vi "GL_controller.VI"(0 "Motion Settings":T1={"No Motion?"=FALSE, "Motion System"=enum."NI 735x", "Motion Bd ID"=1, "Motion Profile"="SMAC1", "# Axis"=1, "Reverse Z axis?"=TRUE, "SMAC Axis"=0, "scan pair"=enum."y-(x) scan", "RT fps"=6.0, "Steps per mm"=[1000, 1000, 1000, 1000], "Motor Parameters"={"velocity ct/s"=[10000.0, 10000.0, 10000.0, 50000.0], "accel ct/s^2"=[50000.0, 50000.0, 50000.0, 200000.0]}, "One Way Scan"=FALSE, "Reverse One Way Scan"=FALSE, "Global Position (mm)"=[], "Plane"=0, "Distance between\nscan lines (um)"=0.0, "Distance between\nscan planes (um)"=0.0, "number of scan planes"=1, "Total steps in line"=0, "Xtra plane\ndistance  (um)"=100, "Xtra planes "=1, "Add Axis"=FALSE, "overshoot cts"=200, "BKPT Shift"=0, "Scan Start Time (ms)"=0, "ESP VISA"="GPIB::1::INSTR", "3rd Axis"=1, "GL Ref Out"=refnum, "Galil Address"=""} {"3rd Axis" items=["x", "y", "z", "w"]; "Xtra planes" min=1; "Xtra plane\ndistance  (um)" min=0; "Distance between\nscan planes (um)" format="%.2f"; "Distance between\nscan lines (um)" format="%.2f"; "SMAC Axis" items=["None"=0, "Axis 1"=1, "Axis 2"=2, "Axis 3"=3, "Axis 4"=4, "Axis 5"=5, "Axis 6"=6, "Axis 7"=7, "Axis 8"=8, "Vector Space 1"=17, "Vector Space 2"=18, "Vector Space 3"=19, "Vector Space 4"=20]; "Motion Bd ID" min=1 max=32 step=1}, 4 "Initialize":bool=TRUE) -> (5 "Motion Settings Out":T1={"No Motion?"=FALSE, "Motion System"=enum."NI 735x", "Motion Bd ID"=1, "Motion Profile"="SMAC1", "# Axis"=1, "Reverse Z axis?"=TRUE, "SMAC Axis"=0, "scan pair"=enum."y-(x) scan", "RT fps"=6.0, "Steps per mm"=[1000, 1000, 1000, 1000], "Motor Parameters"={"velocity ct/s"=[10000.0, 10000.0, 10000.0, 50000.0], "accel ct/s^2"=[50000.0, 50000.0, 50000.0, 200000.0]}, "One Way Scan"=FALSE, "Reverse One Way Scan"=FALSE, "Global Position (mm)"=[], "Plane"=0, "Distance between\nscan lines (um)"=0.0, "Distance between\nscan planes (um)"=0.0, "number of scan planes"=1, "Total steps in line"=0, "Xtra plane\ndistance  (um)"=100, "Xtra planes "=1, "Add Axis"=FALSE, "overshoot cts"=200, "BKPT Shift"=0, "Scan Start Time (ms)"=0, "ESP VISA"="GPIB::1::INSTR", "3rd Axis"=1, "GL Ref Out"=refnum, "Galil Address"=""} {"3rd Axis" items=["x", "y", "z", "w"]; "Xtra planes" min=1; "Xtra plane\ndistance  (um)" min=0; "Distance between\nscan planes (um)" format="%.2f"; "Distance between\nscan lines (um)" format="%.2f"; "SMAC Axis" items=["None"=0, "Axis 1"=1, "Axis 2"=2, "Axis 3"=3, "Axis 4"=4, "Axis 5"=5, "Axis 6"=6, "Axis 7"=7, "Axis 8"=8, "Vector Space 1"=17, "Vector Space 2"=18, "Vector Space 3"=19, "Vector Space 4"=20]; "Motion Bd ID" min=1 max=32 step=1}, 6 "error out":errorcluster)   [LabVIEW 2022 SP3]
uses:
  NI_controller/-NI_MotionRoutines/MotionParameters.ctl
  NI_controller/-NI_MotionRoutines/MotionSys.ctl
  -MotionRoutines/ScanAxis.ctl
  -MotionRoutines/3rdAxis.ctl
  Command Menu.ctl
  GL Axis Control.ctl
  -ScanSystem/Controls/location.ctl
  <vilib>/event_ctls.llb/eventvkey.ctl
  -MotionRoutines/MotionGlobals.vi
panel:
  in  "Cent All":bool
  in  "Position (mm) (Abs)":dbl format="%.3f"
  in  "Axis Tune":enum32{"Axis 1", "Axis 2", "Axis 3", "Axis 4"}(radio)
  in  "Inc. Step\nSize (mm)":dbl=0.5
  out "Found Center":bool
  in  "Cent X":bool
  in  "Cent Y":bool
  in  "Cent Z":bool
  in  "Abs W Pos (mm)":dbl format="%.3f"
  in  "Abs Z Pos (mm)":dbl format="%.3f"
  in  "Abs Y Pos (mm)":dbl format="%.3f"
  in  "Abs X Pos (mm)":dbl format="%.3f"
  in  "Def Abs":bool
  in  "Select V&A":bool
  in  "Slave Axis":u16(ring)=2 items=["Axis 1"=1, "Axis 2"=2, "Axis 3"=3, "Axis 4"=4]
  in  "Master Axis":u16(ring)=1 items=["Axis 1"=1, "Axis 2"=2, "Axis 3"=3, "Axis 4"=4]
  in  "Enable Gearing":bool
  out "Angle":dbl=45.000038009906035
  in  "Ratio Denom":u16=1 min=1 max=32767
  in  "Ratio Num":i16 min=0
  in  "Cent W":bool
  in  "W Position (mm)":dbl format="%.3f"
  in  "FineMi4":bool
  in  "FinePl4":bool
  in  "Rst4":bool
  in  "Ax4Plus":bool
  in  "Ax4Minus":bool
  in  "Z Position (mm)":dbl format="%.3f"
  in  "FineMi3":bool
  in  "FinePl3":bool
  in  "Rst3":bool
  in  "Ax3Plus":bool
  in  "Ax3Minus":bool
  in  "Y Position (mm)":dbl format="%.3f"
  in  "FineMi2":bool
  in  "FinePl2":bool
  in  "Rst2":bool
  in  "Ax2Plus":bool
  in  "Ax2Minus":bool
  in  "X Position (mm)":dbl format="%.3f"
  in  "stop":bool
  in  "FineMi1":bool
  in  "FinePl1":bool
  in  "Rst1":bool
  in  "Ax1Plus":bool
  in  "Ax1Minus":bool
  # "Units are in mm. \"Rst\" zeros the position. Blue circles move 1 cm for linear."
  # "Redefine\nAbs Position"
  # "Be very careful with this mode it is not fully programmed"
  # "X Axis (mm)"
  # "Y Axis  (mm)"
  # "Z Axis (mm)"
  # "LinInd (mm)"
  # "1-D and 2-D B scan settings"
  # "1-D and 2-D B scan settings"
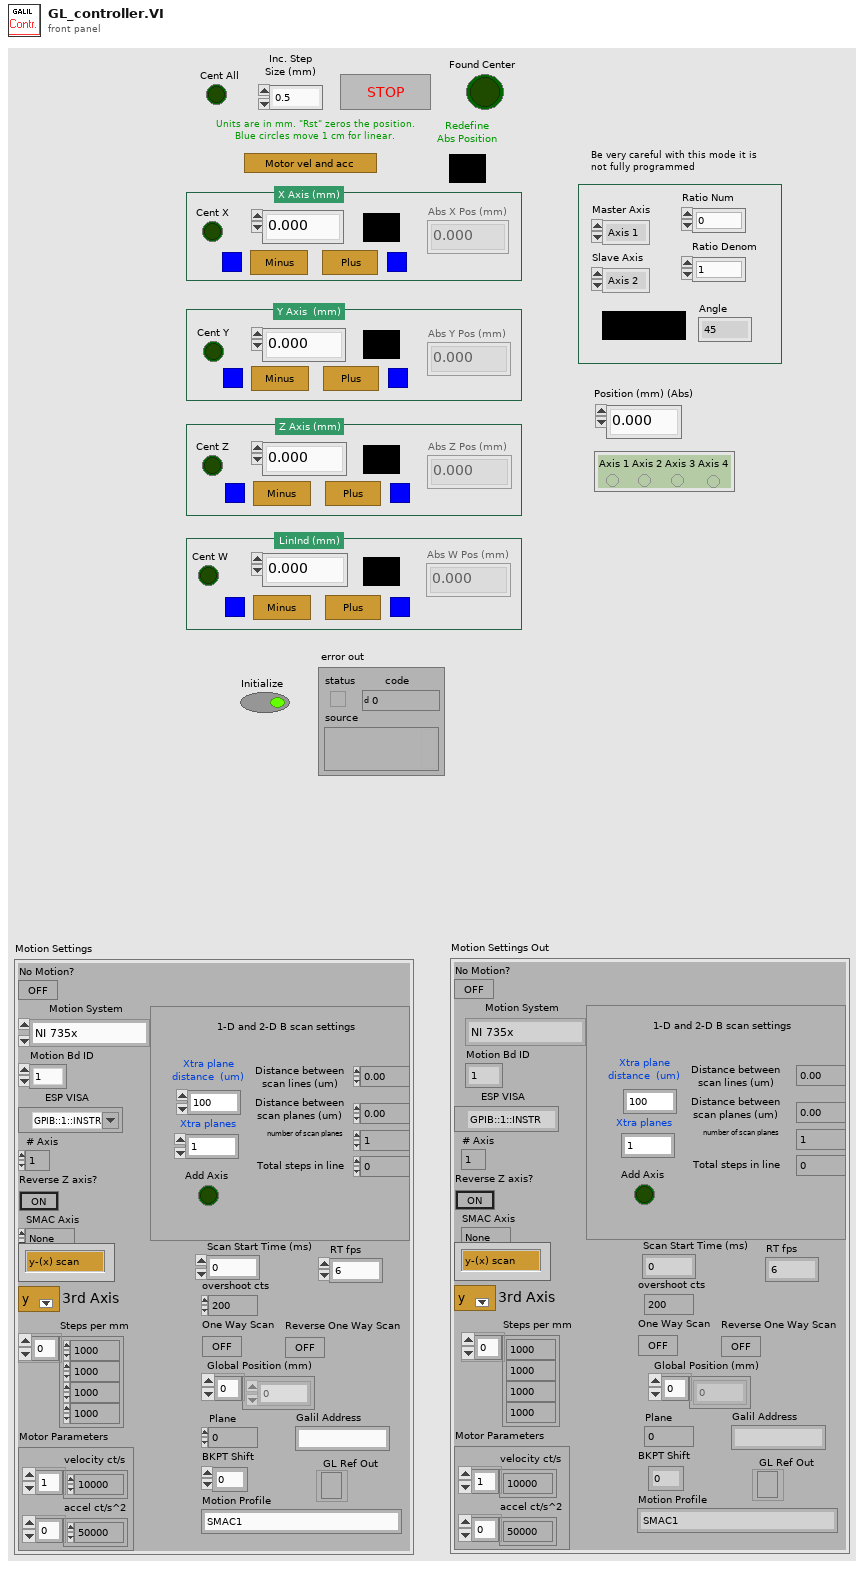
[diagram p1: front panel]
types:
  T1 = typedef "MotionParameters.ctl" = cluster{"No Motion?":bool, "Motion System":T2, "Motion Bd ID":u8, "Motion Profile":string, "# Axis":i8, "Reverse Z axis?":bool, "SMAC Axis":u16, "scan pair":T3, "RT fps":sgl, "Steps per mm":i32[], "Motor Parameters":cluster{"velocity ct/s":dbl[], "accel ct/s^2":dbl[]}, "One Way Scan":bool, "Reverse One Way Scan":bool, "Global Position (mm)":dbl[], "Plane":i32, "Distance between\nscan lines (um)":sgl, "Distance between\nscan planes (um)":sgl, "number of scan planes":i32, "Total steps in line":i32, "Xtra plane\ndistance  (um)":i32, "Xtra planes ":i32, "Add Axis":bool, "overshoot cts":i32, "BKPT Shift":i32, "Scan Start Time (ms)":u32, "ESP VISA":refnum<visa-resource-name>, "3rd Axis":T4, "GL Ref Out":refnum<k7>, "Galil Address":string}
  T2 = typedef "MotionSys.ctl" = enum16{"MM3000", "NI 735x", "Newport ESP", "No Motion Card", "Galil"}
  T3 = typedef "ScanAxis.ctl" = enum16{"y-(x) scan", "x-(y) scan", "z-(x) scan", "z-(y) scan", "y-(z) scan", "x-(z) scan", "w-(x) scan", "w-(y) scan", "w-(z) scan", "x-(w) scan", "y-(w) scan", "z-(w) scan"}
  T4 = typedef "3rdAxis.ctl" = u16
  T5 = typedef "GL Axis Control.ctl" = u16
  T6 = typedef "Command Menu.ctl" = enum16{"CommandPassThrough", "Abort Motion", "Define Pos", "Velocity", "Acceleration", "Deceleration", "Position Rel", "Postion Abs", "Begin Move", "After Move", "Home", "KI", "KD", "KP", "IL", "Config I/O", "Set Bit", "Clear Bit", "Motor Off", "Moto On", "Status", "Execute", "Halt Execute", "HX Status", "Tell Velocity", "Check Motion", "BreakPoint", "Tell Position", "Current Code Line", "Tell Switches", "OC Force On", "OC Off", "Pos Soft Limit", "Rev Soft Limit"}
  T7 = enum8{"Enabled", "Disabled", "Disabled and Grayed Out"}
  T8 = typedef "location.ctl" = enum16{"Automatic", "WCM Main", "Hawaii", "Columbia MM3000", "Columbia  NI System", "NYU", "RRI 2", "UHI Allen", "CUMC RT", "Chiba", "Stony Brook", "WCM Microscopy", "WCM Aeoretch", "WCM Optics Lab", "WCM Main 2Axis", "WCM Rotation", "WCM SAM SMAC", "SERI GP"}
  T9 = cluster{"Steps per mm[0]":i32, "Steps per mm[1]":i32, "Steps per mm[2]":i32, "Steps per mm[3]":i32}
  T10 = enum16{"Absolute Position", "Relative Position", "Velocity", "Relative to Cap Pos", "Modulus Position", "Absolute Contouring", "Relative Contouring"}
  T11 = typedef "eventvkey.ctl" = enum16{"ASCII", "Enter", "Return", "Shift", "Ctrl", "Alt", "Cmd", "Opt", "Caps", "NumLock", "Clear", "Break", "Up", "Down", "Left", "Right", "Insert", "Delete", "Home", "End", "PageUp", "PageDown", "Escape", "Help", "Pause", "ScrollLock", "F1", "F2", "F3", "F4", "F5", "F6", "F7", "F8", "F9", "F10", "F11", "F12", "F13", "F14", "F15", "F16", "F17", "F18", "F19", "F20", "F21", "F22", "F23", "F24", "Play", "VolumeUp", "VolumeDown", "Mute", "Two Byte Char"}
  T12 = cluster{"Shift":bool, "Ctrl":bool, "Alt":bool, "Cmd":bool, "Opt":bool}
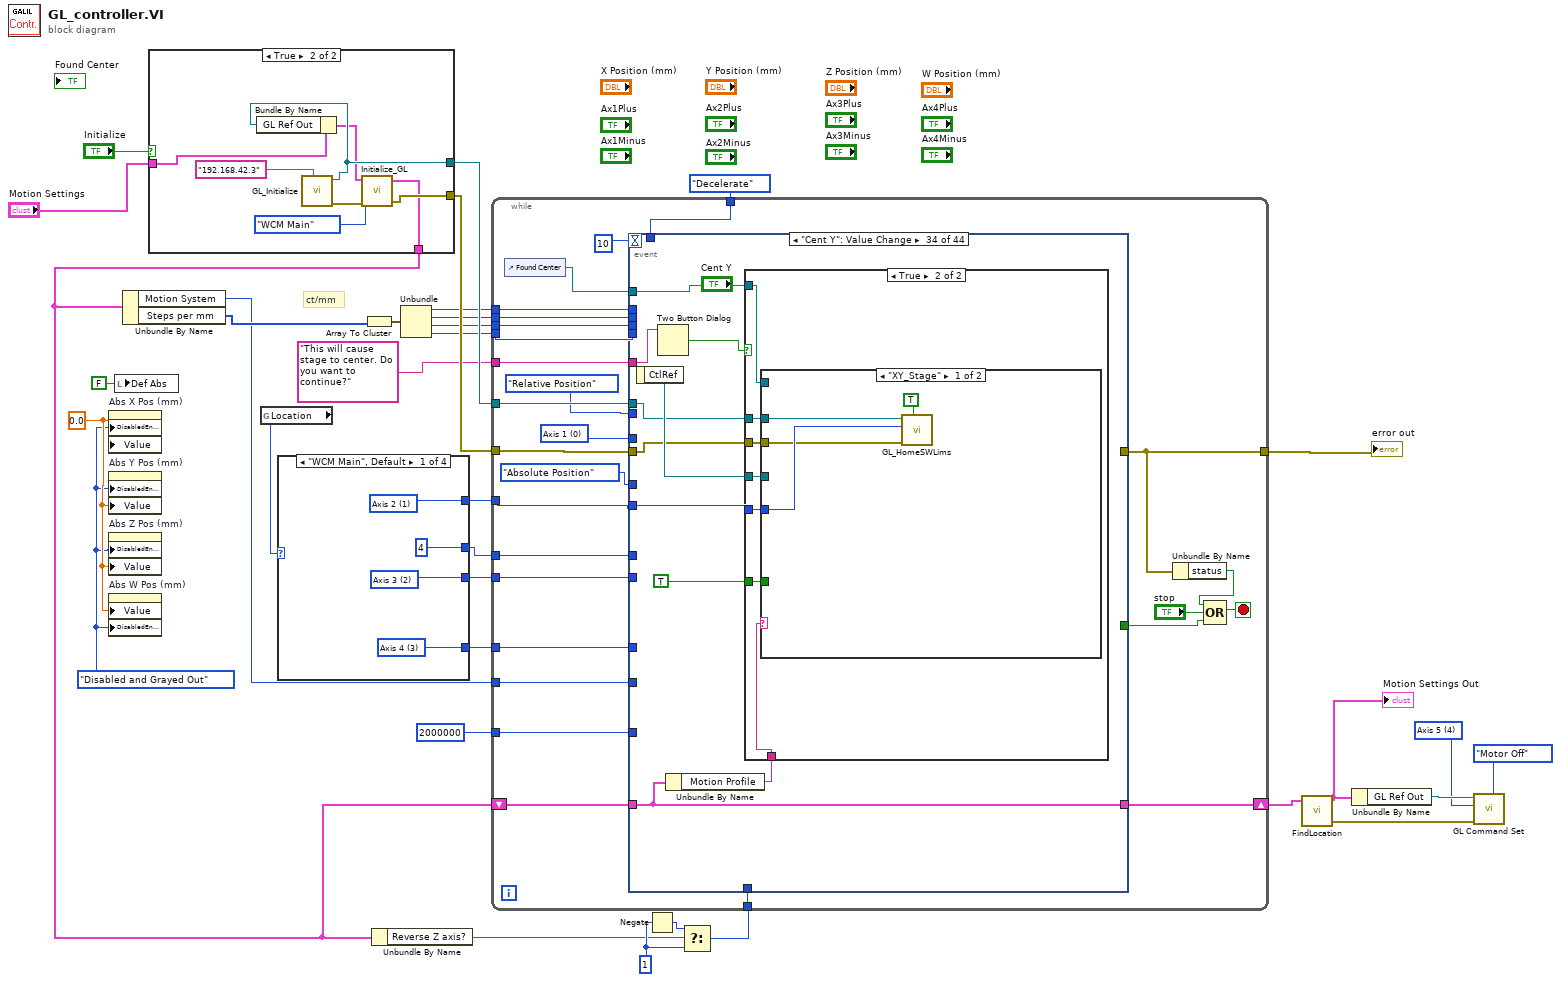
[diagram p0: block diagram]
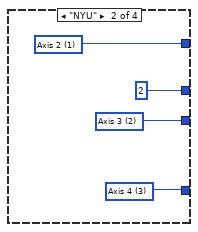
[diagram p2: hidden frame]
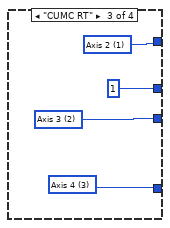
[diagram p3: hidden frame]
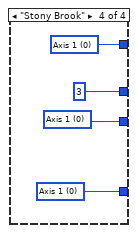
[diagram p4: hidden frame]
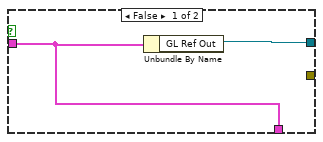
[diagram p5: hidden frame]
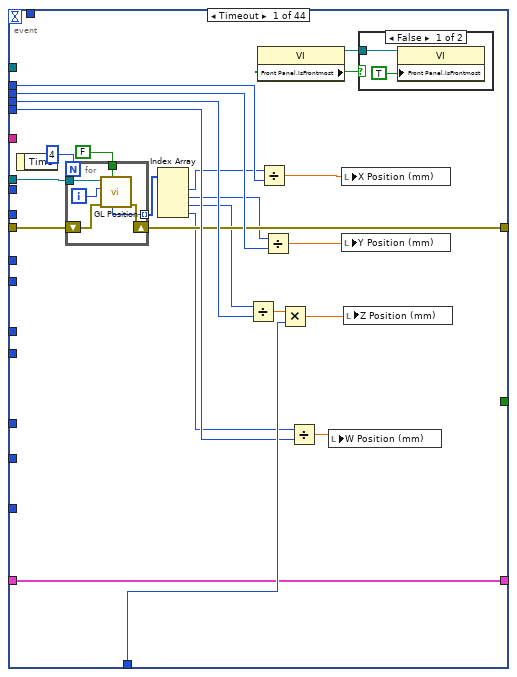
[diagram p6: hidden frame]
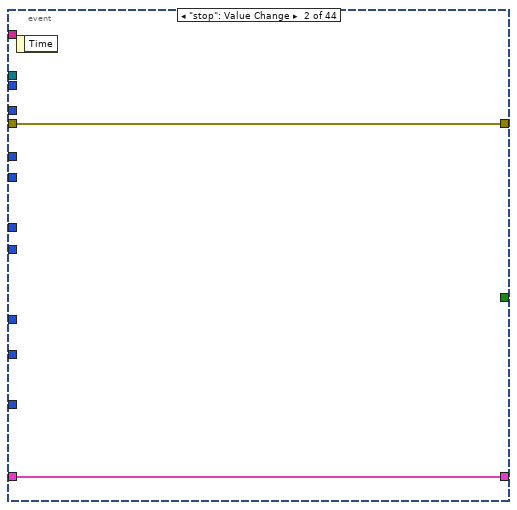
[diagram p8: hidden frame]
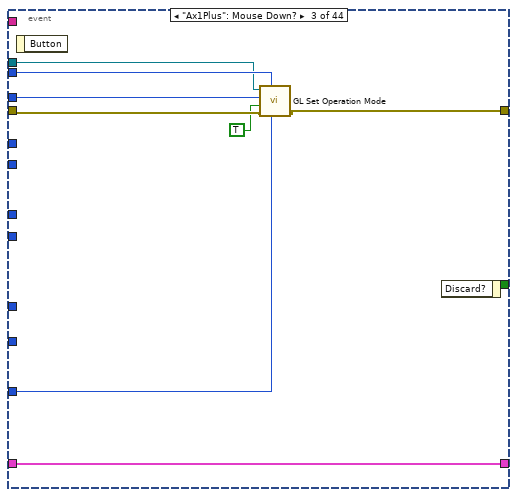
[diagram p9: hidden frame]
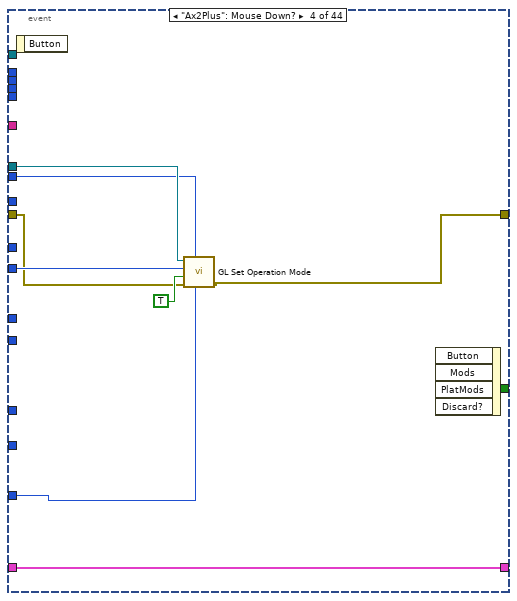
[diagram p10: hidden frame]
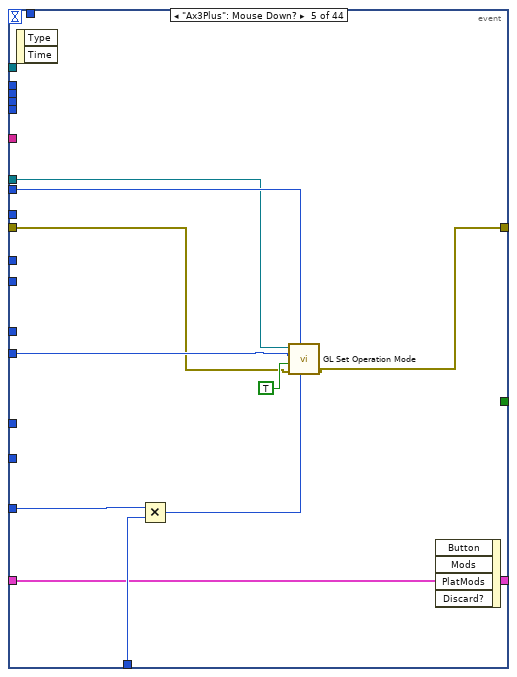
[diagram p11: hidden frame]
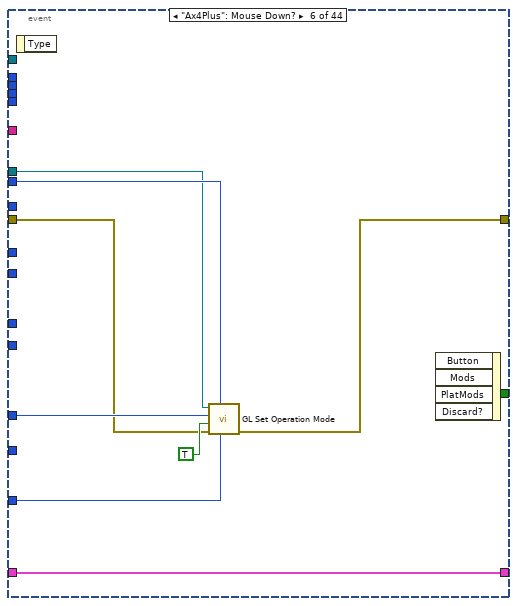
[diagram p12: hidden frame]
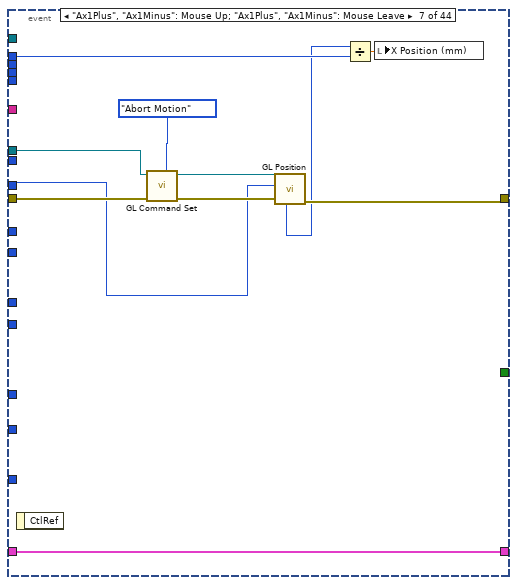
[diagram p13: hidden frame]
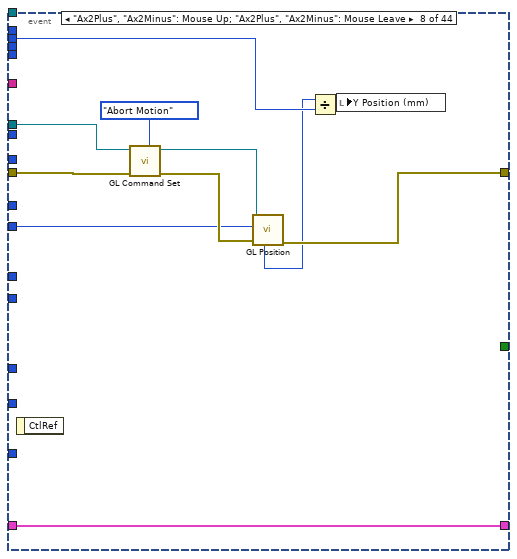
[diagram p14: hidden frame]
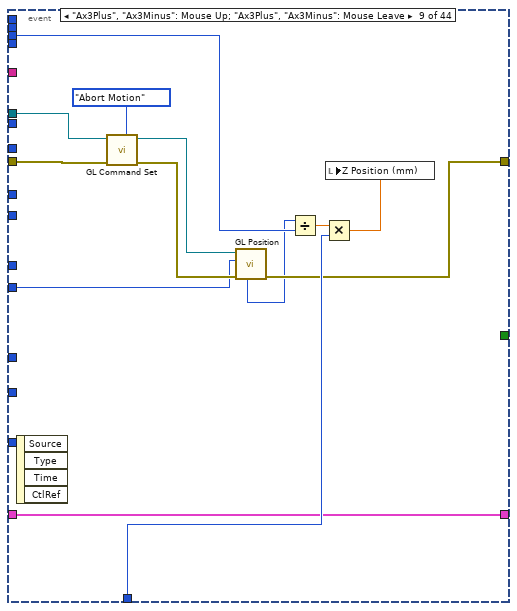
[diagram p15: hidden frame]
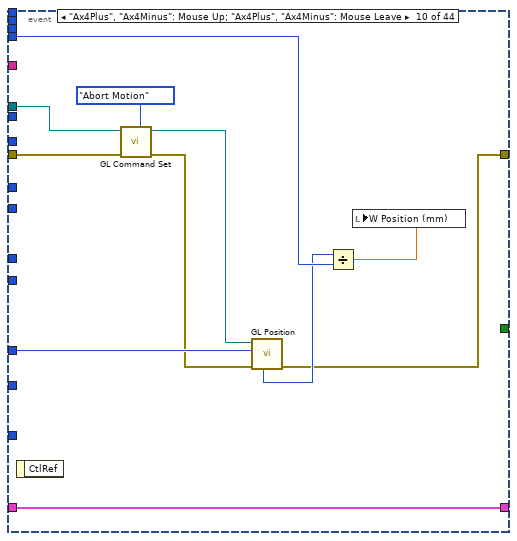
[diagram p16: hidden frame]
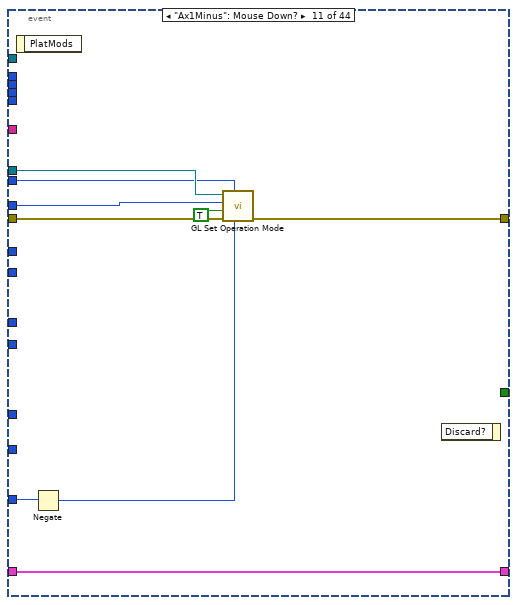
[diagram p17: hidden frame]
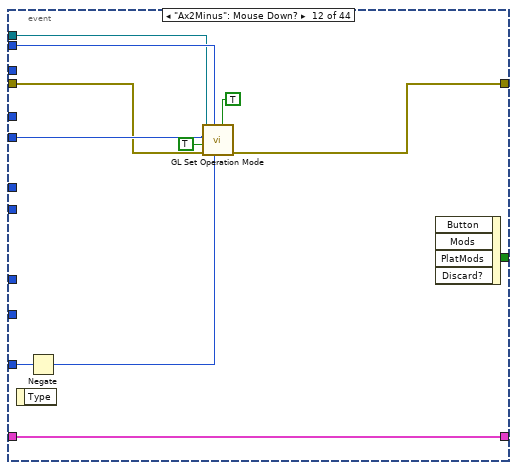
[diagram p18: hidden frame]
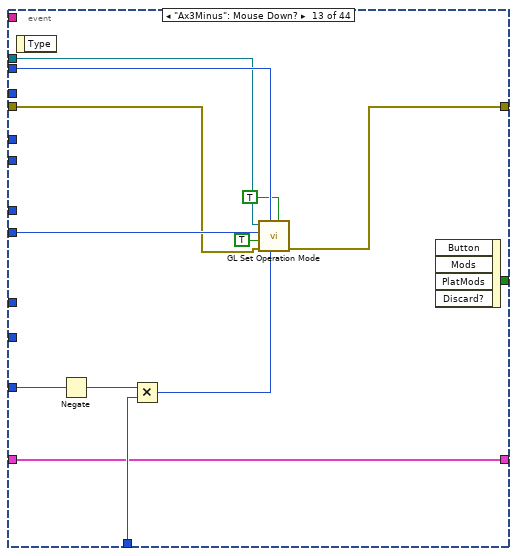
[diagram p19: hidden frame]
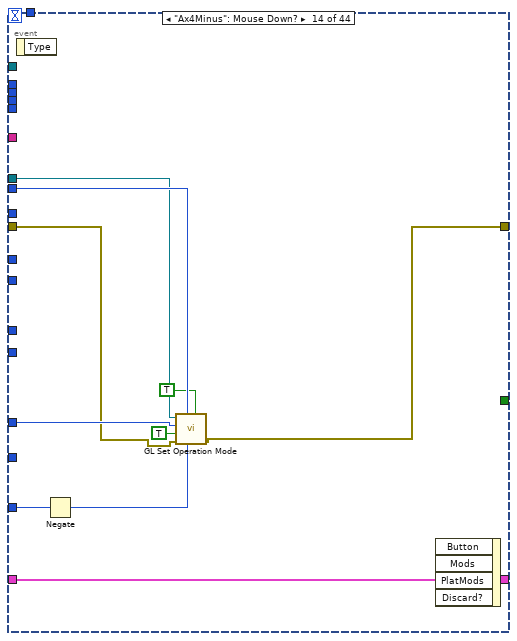
[diagram p20: hidden frame]
diagram:
  w1 = T5 4 items=["Axis 1", "Axis 2", "Axis 3", "Axis 4", "Axis 5", "Axis 6", "Axis 7", "Axis 8"] ("Axis")
  w11 = T7."Disabled and Grayed Out" ("Disabled")
  w17 = 0.0 ("Abs X Pos (mm)")
  w29 = 1
  # "ct/mm"
  n1 = property on="Abs X Pos (mm)" class="DigNum (strict)"("DisabledEnum"=w11, "Value"=w17) -> ()  [unwired: 2 in, 2 out]
  n2 = property on="Abs Y Pos (mm)" class="DigNum (strict)"("DisabledEnum"=w11, "Value"=w17) -> ()  [unwired: 2 in, 2 out]
  n3 = property on="Abs Z Pos (mm)" class="DigNum (strict)"("DisabledEnum"=w11, "Value"=w17) -> ()  [unwired: 2 in, 2 out]
  n4 = property on="Abs W Pos (mm)" class="DigNum (strict)"("Value"=w17, "DisabledEnum"=w11) -> ()  [unwired: 2 in, 2 out]
  n5 = local write "Def Abs"(FALSE ("Visible")) -> ()
  n6 = case shown="True" "Initialize" {
    tunnel: [w36 w40] -> w34
    tunnel: [_ w42] -> w33
    tunnel: "Motion Settings" -> [w35 w41]
    tunnel: [w35 w37] -> w4
    frame False {
      n7 = Unbundle By Name(w35) -> ("GL Ref Out"=w36:refnum<k7>)
    }
    frame True {
      n8 = call "GL_Initialize.vi"("IP Address/COM"="192.168.42.3") -> ("error out"=w43:errorcluster, "GL Ref Out"=w40:refnum<k7>)  [unwired: 5 in, 2 out]
      n9 = Bundle By Name(cluster=w41, "GL Ref Out"=w40) -> (w39:T1)
      n10 = call "Initialize_GL.vi"("Motion Settings"=w39, "Location"=location."WCM Main", "error in"=w43) -> ("Motion Settings"=w37:T1, "error out"=w42:errorcluster)  [unwired: 2 in, 1 out]
    }
  }
  n11 = Unbundle By Name(w4) -> ("Motion System"=w13:T2, "Steps per mm"=w15:i32[])
  n12 = global read "MotionGlobals.vi" "Location"() -> (w25:T8)
  n13 = case shown="\"WCM Main\", Default" w25 {
    tunnel: [w47 w49 w53 w57] -> w27
    tunnel: [w45 w50 w54 w58] -> w26
    tunnel: [4 2 1 3] -> w8
    tunnel: [w46 w51 w55 w59] -> w24
    frame "WCM Main", Default {
      w47 = u16 3 items=["Axis 1", "Axis 2", "Axis 3", "Axis 4", "Axis 5", "Axis 6", "Axis 7", "Axis 8"] ("Axis or Vector Space")
      w45 = u16 2 items=["Axis 1", "Axis 2", "Axis 3", "Axis 4", "Axis 5", "Axis 6", "Axis 7", "Axis 8"] ("Axis or Vector Space")
      w46 = u16 1 items=["Axis 1", "Axis 2", "Axis 3", "Axis 4", "Axis 5", "Axis 6", "Axis 7", "Axis 8"] ("Axis or Vector Space")
    }
    frame "NYU" {
      w49 = u16 3 items=["Axis 1", "Axis 2", "Axis 3", "Axis 4", "Axis 5", "Axis 6", "Axis 7", "Axis 8"] ("Axis or Vector Space")
      w50 = u16 2 items=["Axis 1", "Axis 2", "Axis 3", "Axis 4", "Axis 5", "Axis 6", "Axis 7", "Axis 8"] ("Axis or Vector Space")
      w51 = u16 1 items=["Axis 1", "Axis 2", "Axis 3", "Axis 4", "Axis 5", "Axis 6", "Axis 7", "Axis 8"] ("Axis or Vector Space")
    }
    frame "CUMC RT" {
      w53 = u16 3 items=["Axis 1", "Axis 2", "Axis 3", "Axis 4", "Axis 5", "Axis 6", "Axis 7", "Axis 8"] ("Axis or Vector Space")
      w54 = u16 2 items=["Axis 1", "Axis 2", "Axis 3", "Axis 4", "Axis 5", "Axis 6", "Axis 7", "Axis 8"] ("Axis or Vector Space")
      w55 = u16 1 items=["Axis 1", "Axis 2", "Axis 3", "Axis 4", "Axis 5", "Axis 6", "Axis 7", "Axis 8"] ("Axis or Vector Space")
    }
    frame "Stony Brook" {
      w57 = u16 0 items=["Axis 1", "Axis 2", "Axis 3", "Axis 4", "Axis 5", "Axis 6", "Axis 7", "Axis 8"] ("Axis or Vector Space")
      w58 = u16 0 items=["Axis 1", "Axis 2", "Axis 3", "Axis 4", "Axis 5", "Axis 6", "Axis 7", "Axis 8"] ("Axis or Vector Space")
      w59 = u16 0 items=["Axis 1", "Axis 2", "Axis 3", "Axis 4", "Axis 5", "Axis 6", "Axis 7", "Axis 8"] ("Axis or Vector Space")
    }
  }
  n14 = Array To Cluster(array=w15) -> (cluster=w23:T9)
  n15 = Unbundle By Name(w4) -> ("Reverse Z axis?"=w16:bool)
  n16 = Unbundle(w23) -> ("Steps per mm[0]"=w22:i32, "Steps per mm[1]"=w21:i32, "Steps per mm[2]"=w20:i32, "Steps per mm[3]"=w19:i32)
  n17 = Negate(x=w29) -> (-x=w31:i32)
  n18 = Select(t=w31, s=w16, f=w29) -> (s? t:f=w30:i32)
  n19 = while {
    tunnel: [w82] -> w14
    tunnel: w33 -> [w62]
    tunnel: w34 -> [w69]
    tunnel: w30 -> [w84]
    tunnel: w13 -> [w83]
    tunnel: 2000000 -> [w81]
    tunnel: enum16{"Decelerate", "Halt", "Kill"}."Decelerate" ("Stop Type (Decel)") -> [w80]
    tunnel: w27 -> [w66]
    tunnel: w26 -> [w65]
    tunnel: w24 -> [w64]
    tunnel: w22 -> [w79]
    tunnel: w21 -> [w78]
    tunnel: w20 -> [w77]
    tunnel: w19 -> [w76]
    shift-right: [w74] -> w10
    shift-left: w4 -> [w75]
    tunnel: "This will cause stage to center. Do you want to continue?" ("message") -> [w70]
    tunnel: w8 -> [w67]
    stop <- w86 stop-if-true
    w63 = u16 0 items=["Axis 1", "Axis 2", "Axis 3", "Axis 4", "Axis 5", "Axis 6", "Axis 7", "Axis 8"] ("Axis or Vector Space")
    n20 = control-ref of="Found Center"() -> (w72:refnum<vi>)
    n21 = event shown="[33] \"Cent Y\": Value Change" {
      selector: _ -> [_ _ _ _ _ _ _ _ _ _ _ _ _ _ _ _ _ _ _ _ _ _ _ _ _ _ _ _ _ _ _ _ _ _ _ _ _ _ _ _ _ _ _ _]
      dyn-events: _ -> [_ _ _ _ _ _ _ _ _ _ _ _ _ _ _ _ _ _ _ _ _ _ _ _ _ _ _ _ _ _ _ _ _ _ _ _ _ _ _ _ _ _ _ _]
      timeout: 10 -> [_ _ _ _ _ _ _ _ _ _ _ _ _ _ _ _ _ _ _ _ _ _ _ _ _ _ _ _ _ _ _ _ _ _ _ _ _ _ _ _ _ _ _ _]
      tunnel: w62 -> [w97 w120 w126 w129 w138 w147 w159 w168 w182 w195 w202 w211 w222 w233 w246 w249 w257 w266 w274 w279 w289 w299 w312 w317 w327 w337 w351 w358 w382 w389 w399 _ w455 w480 _ w538 w547 _ _ _ w585 w591 w599 w613]
      tunnel: w80 -> [_ _ _ _ _ _ _ _ _ _ _ _ _ _ _ _ _ _ _ _ _ _ _ _ _ _ _ _ _ _ _ _ _ _ _ _ _ _ _ _ _ _ _ _]
      tunnel: w63 -> [_ _ w123 _ _ _ w155 _ _ _ w206 _ _ _ w245 _ _ _ w270 _ _ _ w309 _ _ _ w349 _ _ _ _ _ w451 _ _ _ _ _ _ _ w584 _ _ _]
      tunnel: w64 -> [_ _ _ w130 _ _ _ w167 _ _ _ w216 _ _ _ w253 _ _ _ w280 _ _ _ w318 _ _ _ w363 _ _ _ _ _ w489 _ _ _ _ _ _ _ w593 _ _]
      tunnel: w65 -> [_ _ _ _ w141 _ _ _ w180 _ _ _ w225 _ _ _ w258 _ _ _ w292 _ _ _ w328 _ _ _ w380 _ _ _ _ _ w519 _ _ _ _ _ _ _ w603 _]
      tunnel: w66 -> [_ _ _ _ _ w149 _ _ _ w194 _ _ _ w236 _ _ _ w263 _ _ _ w300 _ _ _ w338 _ _ _ w394 _ _ _ _ _ w539 _ _ _ _ _ _ _ w610]
      tunnel: [w96 w120 w127 w134 w143 w152 w160 w171 w181 w190 w204 w217 w228 w239 w247 w252 w260 _ w275 w284 w294 w304 w313 w322 w332 w342 w350 w364 w383 w390 w404 _ _ _ _ _ _ _ _ _ w586 w592 w600 w614] -> w82
      tunnel: [_ _ _ _ _ _ _ _ _ _ _ _ _ _ _ _ _ w267 _ _ _ _ _ _ _ _ _ _ _ _ _ _ _ _ _ _ _ _ _ _ _ _ _ _] -> _
      tunnel: w84 -> [w106 _ _ _ w146 _ _ _ w187 _ _ _ w231 _ _ _ _ _ _ _ w298 _ _ _ w336 _ _ _ w386 _ _ _ _ _ _ _ _ _ _ _ _ _ w607 _]
      tunnel: w83 -> [_ _ _ _ _ _ _ _ _ _ _ _ _ _ _ _ _ _ _ _ _ _ _ _ _ _ _ _ _ _ _ _ _ _ _ _ _ _ _ _ _ _ _ _]
      tunnel: w81 -> [_ _ w124 w133 w145 w151 _ _ _ _ w209 w219 w229 w241 _ _ _ _ _ _ _ _ _ _ _ _ _ _ _ _ _ _ _ _ _ _ _ _ _ _ _ _ _ _]
      tunnel: w79 -> [w103 _ _ _ _ _ w164 _ _ _ _ _ _ _ _ _ _ _ w278 _ _ _ w316 _ _ _ w355 _ _ _ _ _ _ _ _ _ _ _ _ _ w590 _ _ _]
      tunnel: w78 -> [w102 _ _ _ _ _ _ w175 _ _ _ _ _ _ _ _ _ _ _ w287 _ _ _ w325 _ _ _ w367 _ _ _ _ _ _ _ _ _ _ _ _ _ w598 _ _]
      tunnel: w77 -> [w101 _ _ _ _ _ _ _ w186 _ _ _ _ _ _ _ _ _ _ _ w297 _ _ _ w335 _ _ _ w385 _ _ _ _ _ _ _ _ _ _ _ _ _ w609 _]
      tunnel: w76 -> [w100 _ _ _ _ _ _ _ _ w199 _ _ _ _ _ _ _ _ _ _ _ w307 _ _ _ w345 _ _ _ w397 _ _ _ _ _ _ _ _ _ _ _ _ _ w618]
      tunnel: w75 -> [w99 w119 w128 w136 w137 w154 w163 w174 w177 w198 w208 w218 w220 w240 w248 w255 w262 w269 w277 w286 w288 w306 w315 w324 w326 w344 w354 w366 w373 w396 w402 w422 w450 w483 w513 w533 w551 w571 w576 w579 w588 w596 w605 w616]
      tunnel: [w99 w119 w128 w136 w137 w154 w163 w174 w177 w198 w208 w218 w220 w240 w248 w255 w262 w269 w277 w286 w288 w306 w315 w324 w326 w344 w354 w366 w373 w396 w400 w422 w450 w483 w513 w533 w551 w571 w576 w579 w588 w596 w605 w616] -> w74
      tunnel: w72 -> [_ _ _ _ _ _ _ _ _ _ _ _ _ _ _ _ _ _ _ _ _ _ _ _ _ _ _ _ _ _ _ _ w454 w486 w517 w543 w552 _ _ _ _ _ _ _]
      tunnel: [_ _ _ _ _ _ _ _ _ _ _ _ _ _ _ _ _ _ _ _ _ _ _ _ _ _ _ _ _ _ _ w420 _ _ _ _ _ _ _ _ _ _ _ _] -> w71
      tunnel: w70 -> [_ _ _ _ _ _ _ _ _ _ _ _ _ _ _ _ _ _ _ _ _ _ _ _ _ _ _ _ _ _ _ _ w453 w485 w515 _ _ _ _ _ _ _ _ _]
      tunnel: T10."Absolute Position" ("Position Mode (Absolute)") -> [_ _ _ _ _ _ _ _ _ _ _ _ _ _ _ _ _ _ _ _ _ _ _ _ _ _ w346 w359 _ w391 _ _ _ _ _ _ _ _ _ _ _ _ _ _]
      tunnel: w69 -> [w98 _ w122 w132 w139 w148 w158 w169 w178 w196 w205 w213 w226 w235 w244 w250 w259 w264 w272 w282 w290 w301 w310 w320 w329 w339 w348 w360 w377 w392 w401 _ w448 w481 w514 w540 w549 _ _ _ w582 _ w601 w611]
      tunnel: T10."Relative Position" ("Position Mode (Absolute)") -> [_ _ w125 w131 w140 w150 _ _ _ _ w201 w214 w227 w238 _ _ _ _ w271 w281 w291 w302 w308 w319 w330 w340 _ _ w371 _ _ _ _ _ _ _ _ _ _ _ _ _ _ _]
      tunnel: w67 -> [_ _ _ _ _ _ _ _ _ _ _ _ _ _ _ _ _ _ _ _ _ _ _ _ _ _ _ _ _ _ _ _ _ _ _ _ w548 _ _ _ _ _ _ _]
      event Timeout {
        n22 = event-data() -> ()  [unwired: 2 out]
        n23 = for {
          N: 4 -> [_]
          tunnel: w98 -> [w116]
          tunnel: FALSE ("Wait for Motion Complete") -> [w113]
          shift-right: [w114] -> w96
          shift-left: w97 -> [w115]
          tunnel: [w112] -> w88 mode=indexing
          i -> [w111]
          n24 = call "GL Position.vi"("Wait for Motion Complete"=w113, "error in (no error)"=w115, "Axis"=w111, "Galil.IGalil"=w116) -> ("error out"=w114:errorcluster, "Axis Position"=w112:i32)  [unwired: 2 in, 2 out]
        }
        n25 = Index Array(array=w88) -> (element #1=w94:i32, element #2=w93:i32, element #3=w92:i32, element #4=w91:i32)  [unwired: 4 in]
        n26 = Divide(x=w92, y=w101) -> (x/y=w107:dbl)
        n27 = property class="VI"() -> (reference out=w105:refnum<vi>, "Front Panel.IsFrontmost"=w104:bool)  [unwired: 2 in, 1 out]
        n28 = Divide(x=w94, y=w103) -> (x/y=w110:dbl)
        n29 = Divide(x=w93, y=w102) -> (x/y=w109:dbl)
        n30 = Multiply(x=w107, y=w106) -> (x*y=w108:dbl)
        n31 = Divide(x=w91, y=w100) -> (x/y=w95:dbl)
        n32 = local write "W Position (mm)"(w95) -> ()
        n33 = local write "X Position (mm)"(w110) -> ()
        n34 = local write "Y Position (mm)"(w109) -> ()
        n35 = local write "Z Position (mm)"(w108) -> ()
        n36 = case shown="False" w104 {
          tunnel: w105 -> [w118 _]
          frame False {
            n37 = property class="VI"(reference=w118, "Front Panel.IsFrontmost"=TRUE) -> ()  [unwired: 1 in, 2 out]
          }
          frame True {
          }
        }
      }
      event "stop": Value Change {
        n38 = event-data() -> ()  [unwired: 2 out]
      }
      event "Ax1Plus": Mouse Down? {
        n39 = event-data() -> ()  [unwired: 2 out]
        n40 = call "GL Set Operation Mode.vi"("position cts (abs/rel)"=w124, "Position Mode (Absolute)"=w125, "error in (no error)"=w126, "Start Now?"=TRUE, "Axis"=w123, "Galil.IGalil"=w122) -> ("error out"=w127:errorcluster)  [unwired: 3 in, 2 out]
        n41 = event-data() -> ()  [unwired: 1 in, 2 out]
      }
      event "Ax2Plus": Mouse Down? {
        n42 = event-data() -> ()  [unwired: 2 out]
        n43 = call "GL Set Operation Mode.vi"("position cts (abs/rel)"=w133, "Position Mode (Absolute)"=w131, "error in (no error)"=w129, "Start Now?"=TRUE, "Axis"=w130, "Galil.IGalil"=w132) -> ("error out"=w134:errorcluster)  [unwired: 3 in, 2 out]
        n44 = event-data() -> ()  [unwired: 1 in, 5 out]
      }
      event "Ax3Plus": Mouse Down? {
        n45 = event-data() -> ()  [unwired: 3 out]
        n46 = Multiply(x=w145, y=w146) -> (x*y=w142:i32)
        n47 = call "GL Set Operation Mode.vi"("position cts (abs/rel)"=w142, "Position Mode (Absolute)"=w140, "error in (no error)"=w138, "Start Now?"=TRUE, "Axis"=w141, "Galil.IGalil"=w139) -> ("error out"=w143:errorcluster)  [unwired: 3 in, 2 out]
        n48 = event-data() -> ()  [unwired: 1 in, 5 out]
      }
      event "Ax4Plus": Mouse Down? {
        n49 = event-data() -> ()  [unwired: 2 out]
        n50 = call "GL Set Operation Mode.vi"("position cts (abs/rel)"=w151, "Position Mode (Absolute)"=w150, "error in (no error)"=w147, "Start Now?"=TRUE, "Axis"=w149, "Galil.IGalil"=w148) -> ("error out"=w152:errorcluster)  [unwired: 3 in, 2 out]
        n51 = event-data() -> ()  [unwired: 1 in, 5 out]
      }
      event "Ax1Plus", "Ax1Minus": Mouse Up; "Ax1Plus", "Ax1Minus": Mouse Leave {
        n52 = event-data() -> ()  [unwired: 2 out]
        n53 = call "GL Command Set.vi"("Command"=Command_Menu."Abort Motion", "error in (no error)"=w159, "Galil.IGalil"=w158) -> ("error out"=w162:errorcluster, "ref out"=w161:refnum<k7>)  [unwired: 4 in, 3 out]
        n54 = call "GL Position.vi"("error in (no error)"=w162, "Axis"=w155, "Galil.IGalil"=w161) -> ("error out"=w160:errorcluster, "Axis Position"=w156:i32)  [unwired: 3 in, 2 out]
        n55 = Divide(x=w156, y=w164) -> (x/y=w165:dbl)
        n56 = local write "X Position (mm)"(w165) -> ()
      }
      event "Ax2Plus", "Ax2Minus": Mouse Up; "Ax2Plus", "Ax2Minus": Mouse Leave {
        n57 = event-data() -> ()  [unwired: 2 out]
        n58 = call "GL Command Set.vi"("Command"=Command_Menu."Abort Motion", "error in (no error)"=w168, "Galil.IGalil"=w169) -> ("error out"=w173:errorcluster, "ref out"=w172:refnum<k7>)  [unwired: 4 in, 3 out]
        n59 = call "GL Position.vi"("error in (no error)"=w173, "Axis"=w167, "Galil.IGalil"=w172) -> ("error out"=w171:errorcluster, "Axis Position"=w166:i32)  [unwired: 3 in, 2 out]
        n60 = Divide(x=w166, y=w175) -> (x/y=w176:dbl)
        n61 = local write "Y Position (mm)"(w176) -> ()
      }
      event "Ax3Plus", "Ax3Minus": Mouse Up; "Ax3Plus", "Ax3Minus": Mouse Leave {
        n62 = event-data() -> ()  [unwired: 5 out]
        n63 = call "GL Command Set.vi"("Command"=Command_Menu."Abort Motion", "error in (no error)"=w182, "Galil.IGalil"=w178) -> ("error out"=w184:errorcluster, "ref out"=w183:refnum<k7>)  [unwired: 4 in, 3 out]
        n64 = call "GL Position.vi"("error in (no error)"=w184, "Axis"=w180, "Galil.IGalil"=w183) -> ("error out"=w181:errorcluster, "Axis Position"=w179:i32)  [unwired: 3 in, 2 out]
        n65 = Divide(x=w179, y=w186) -> (x/y=w189:dbl)
        n66 = Multiply(x=w189, y=w187) -> (x*y=w188:dbl)
        n67 = local write "Z Position (mm)"(w188) -> ()
      }
      event "Ax4Plus", "Ax4Minus": Mouse Up; "Ax4Plus", "Ax4Minus": Mouse Leave {
        n68 = event-data() -> ()  [unwired: 2 out]
        n69 = call "GL Command Set.vi"("Command"=Command_Menu."Abort Motion", "error in (no error)"=w195, "Galil.IGalil"=w196) -> ("error out"=w192:errorcluster, "ref out"=w191:refnum<k7>)  [unwired: 4 in, 3 out]
        n70 = call "GL Position.vi"("error in (no error)"=w192, "Axis"=w194, "Galil.IGalil"=w191) -> ("error out"=w190:errorcluster, "Axis Position"=w193:i32)  [unwired: 3 in, 2 out]
        n71 = Divide(x=w193, y=w199) -> (x/y=w200:dbl)
        n72 = local write "W Position (mm)"(w200) -> ()
      }
      event "Ax1Minus": Mouse Down? {
        n73 = event-data() -> ()  [unwired: 2 out]
        n74 = Negate(x=w209) -> (-x=w203:i32)
        n75 = call "GL Set Operation Mode.vi"("position cts (abs/rel)"=w203, "Position Mode (Absolute)"=w201, "error in (no error)"=w202, "Start Now?"=TRUE, "Axis"=w206, "Galil.IGalil"=w205) -> ("error out"=w204:errorcluster)  [unwired: 3 in, 2 out]
        n76 = event-data() -> ()  [unwired: 1 in, 2 out]
      }
      event "Ax2Minus": Mouse Down? {
        n77 = event-data() -> ()  [unwired: 2 out]
        n78 = Negate(x=w219) -> (-x=w215:i32)
        n79 = call "GL Set Operation Mode.vi"("LimitWarning?"=TRUE, "position cts (abs/rel)"=w215, "Position Mode (Absolute)"=w214, "error in (no error)"=w211, "Start Now?"=TRUE, "Axis"=w216, "Galil.IGalil"=w213) -> ("error out"=w217:errorcluster)  [unwired: 2 in, 2 out]
        n80 = event-data() -> ()  [unwired: 1 in, 5 out]
      }
      event "Ax3Minus": Mouse Down? {
        n81 = event-data() -> ()  [unwired: 2 out]
        n82 = Negate(x=w229) -> (-x=w230:i32)
        n83 = Multiply(x=w230, y=w231) -> (x*y=w224:i32)
        n84 = call "GL Set Operation Mode.vi"("LimitWarning?"=TRUE, "position cts (abs/rel)"=w224, "Position Mode (Absolute)"=w227, "error in (no error)"=w222, "Start Now?"=TRUE, "Axis"=w225, "Galil.IGalil"=w226) -> ("error out"=w228:errorcluster)  [unwired: 2 in, 2 out]
        n85 = event-data() -> ()  [unwired: 1 in, 5 out]
      }
      event "Ax4Minus": Mouse Down? {
        n86 = event-data() -> ()  [unwired: 2 out]
        n87 = Negate(x=w241) -> (-x=w237:i32)
        n88 = call "GL Set Operation Mode.vi"("LimitWarning?"=TRUE, "position cts (abs/rel)"=w237, "Position Mode (Absolute)"=w238, "error in (no error)"=w233, "Start Now?"=TRUE, "Axis"=w236, "Galil.IGalil"=w235) -> ("error out"=w239:errorcluster)  [unwired: 2 in, 2 out]
        n89 = event-data() -> ()  [unwired: 1 in, 5 out]
      }
      event "Rst1": Value Change {
        w242 = 0 ("Primary Reset Position (0)")
        n90 = event-data() -> ()  [unwired: 3 out]
        n91 = call "GL Command Set.vi"("Command"=Command_Menu."Define Pos", "error in (no error)"=w246, "Value"=w242, "Axis"=w245, "Galil.IGalil"=w244) -> ("error out"=w247:errorcluster)  [unwired: 2 in, 4 out]
        n92 = local write "X Position (mm)"(w242) -> ()
      }
      event "Rst2": Value Change {
        w251 = 0 ("Primary Reset Position (0)")
        n93 = event-data() -> ()  [unwired: 4 out]
        n94 = local write "Y Position (mm)"(w251) -> ()
        n95 = call "GL Command Set.vi"("Command"=Command_Menu."Define Pos", "error in (no error)"=w249, "Value"=w251, "Axis"=w253, "Galil.IGalil"=w250) -> ("error out"=w252:errorcluster)  [unwired: 2 in, 4 out]
      }
      event "Rst3": Value Change {
        w256 = 0 ("Primary Reset Position (0)")
        n96 = event-data() -> ()  [unwired: 4 out]
        n97 = local write "Z Position (mm)"(w256) -> ()
        n98 = call "GL Command Set.vi"("Command"=Command_Menu."Define Pos", "error in (no error)"=w257, "Value"=w256, "Axis"=w258, "Galil.IGalil"=w259) -> ("error out"=w260:errorcluster)  [unwired: 2 in, 4 out]
      }
      event "Rst4": Value Change {
        w265 = 0 ("Primary Reset Position (0)")
        n99 = event-data() -> ()  [unwired: 3 out]
        n100 = local write "W Position (mm)"(w265) -> ()
        n101 = call "GL Command Set.vi"("Command"=Command_Menu."Define Pos", "error in (no error)"=w266, "Value"=w265, "Axis"=w263, "Galil.IGalil"=w264) -> ("error out"=w267:errorcluster)  [unwired: 2 in, 4 out]
      }
      event "FinePl1": Value Change {
        # "# of counts for 1cm"
        n102 = event-data() -> ()  [unwired: 2 out]
        n103 = expression code="x*10"(w278) -> (w273:i32)
        n104 = call "GL Set Operation Mode.vi"("position cts (abs/rel)"=w273, "Position Mode (Absolute)"=w271, "error in (no error)"=w274, "Start Now?"=TRUE, "Axis"=w270, "Galil.IGalil"=w272) -> ("error out"=w275:errorcluster)  [unwired: 3 in, 2 out]
      }
      event "FinePl2": Value Change {
        # "# of counts for 1cm"
        n105 = event-data() -> ()  [unwired: 2 out]
        n106 = expression code="x*10"(w287) -> (w283:i32)
        n107 = call "GL Set Operation Mode.vi"("position cts (abs/rel)"=w283, "Position Mode (Absolute)"=w281, "error in (no error)"=w279, "Start Now?"=TRUE, "Axis"=w280, "Galil.IGalil"=w282) -> ("error out"=w284:errorcluster)  [unwired: 3 in, 2 out]
      }
      event "FinePl3": Value Change {
        # "# of counts for 1cm"
        n108 = event-data() -> ()  [unwired: 2 out]
        n109 = expression code="x*10"(w297) -> (w296:i32)
        n110 = Multiply(x=w296, y=w298) -> (x*y=w293:i32)
        n111 = call "GL Set Operation Mode.vi"("position cts (abs/rel)"=w293, "Position Mode (Absolute)"=w291, "error in (no error)"=w289, "Start Now?"=TRUE, "Axis"=w292, "Galil.IGalil"=w290) -> ("error out"=w294:errorcluster)  [unwired: 3 in, 2 out]
      }
      event "FinePl4": Value Change {
        # "# of counts for 1cm"
        n112 = event-data() -> ()  [unwired: 2 out]
        n113 = expression code="x*10"(w307) -> (w303:i32)
        n114 = call "GL Set Operation Mode.vi"("position cts (abs/rel)"=w303, "Position Mode (Absolute)"=w302, "error in (no error)"=w299, "Start Now?"=TRUE, "Axis"=w300, "Galil.IGalil"=w301) -> ("error out"=w304:errorcluster)  [unwired: 3 in, 2 out]
      }
      event "FineMi1": Value Change {
        # "# of counts for 1cm"
        n115 = event-data() -> ()  [unwired: 4 out]
        n116 = expression code="x*-10"(w316) -> (w311:i32)
        n117 = call "GL Set Operation Mode.vi"("position cts (abs/rel)"=w311, "Position Mode (Absolute)"=w308, "error in (no error)"=w312, "Start Now?"=TRUE, "Axis"=w309, "Galil.IGalil"=w310) -> ("error out"=w313:errorcluster)  [unwired: 3 in, 2 out]
      }
      event "FineMi2": Value Change {
        # "# of counts for 1cm"
        n118 = event-data() -> ()  [unwired: 4 out]
        n119 = expression code="x*-10"(w325) -> (w321:i32)
        n120 = call "GL Set Operation Mode.vi"("position cts (abs/rel)"=w321, "Position Mode (Absolute)"=w319, "error in (no error)"=w317, "Start Now?"=TRUE, "Axis"=w318, "Galil.IGalil"=w320) -> ("error out"=w322:errorcluster)  [unwired: 3 in, 2 out]
      }
      event "FineMi3": Value Change {
        # "# of counts for 1cm"
        n121 = event-data() -> ()  [unwired: 2 out]
        n122 = expression code="x*-10"(w335) -> (w334:i32)
        n123 = Multiply(x=w334, y=w336) -> (x*y=w331:i32)
        n124 = call "GL Set Operation Mode.vi"("position cts (abs/rel)"=w331, "Position Mode (Absolute)"=w330, "error in (no error)"=w327, "Start Now?"=TRUE, "Axis"=w328, "Galil.IGalil"=w329) -> ("error out"=w332:errorcluster)  [unwired: 3 in, 2 out]
      }
      event "FineMi4": Value Change {
        # "# of counts for 1cm"
        n125 = event-data() -> ()  [unwired: 2 out]
        n126 = expression code="x*-10"(w345) -> (w341:i32)
        n127 = call "GL Set Operation Mode.vi"("position cts (abs/rel)"=w341, "Position Mode (Absolute)"=w340, "error in (no error)"=w337, "Start Now?"=TRUE, "Axis"=w338, "Galil.IGalil"=w339) -> ("error out"=w342:errorcluster)  [unwired: 3 in, 2 out]
      }
      event "X Position (mm)": Value Change {
        n128 = event-data() -> ("NewVal"=w356:dbl)  [unwired: 1 out]
        n129 = Multiply(x=w356, y=w355) -> (x*y=w352:dbl)
        n130 = Subtract(x=w352, y=0.0) -> (x-y=w357:dbl)
        n131 = To Long Integer(number=w357) -> ()  [unwired: 1 out]
        n132 = call "GL Set Operation Mode.vi"("position cts (abs/rel)"=w352, "Position Mode (Absolute)"=w346, "error in (no error)"=w351, "Start Now?"=TRUE, "Axis"=w349, "Galil.IGalil"=w348) -> ("error out"=w350:errorcluster)  [unwired: 3 in, 2 out]
      }
      event "Y Position (mm)": Value Change {
        n133 = event-data() -> ("NewVal"=w368:dbl)  [unwired: 1 out]
        n134 = Multiply(x=w368, y=w367) -> (x*y=w361:dbl)
        n135 = Subtract(x=w361, y=0.0) -> (x-y=w369:dbl)
        n136 = To Long Integer(number=w369) -> ()  [unwired: 1 out]
        n137 = call "GL Set Operation Mode.vi"("position cts (abs/rel)"=w361, "Position Mode (Absolute)"=w359, "error in (no error)"=w358, "Start Now?"=TRUE, "Axis"=w363, "Galil.IGalil"=w360) -> ("error out"=w364:errorcluster)  [unwired: 3 in, 2 out]
      }
      event "Z Position (mm)": Value Change {
        n138 = event-data() -> ("NewVal"=w387:dbl)  [unwired: 1 out]
        n139 = Compound Arithmetic op=MULTIPLY(w387, w385, w386) -> (w372:dbl)
        n140 = call "GL Command Set.vi"("Command"=Command_Menu."Tell Position", "error in (no error)"=w382, "Axis"=w380, "Galil.IGalil"=w377) -> ("error out"=w381:errorcluster, "Response#"=w379:i32, "Axis Out"=w375:T5, "ref out"=w376:refnum<k7>)  [unwired: 3 in, 1 out]
        n141 = Subtract(x=w372, y=w379) -> (x-y=w370:dbl)
        n142 = To Long Integer(number=w370) -> (32bit integer=w378:i32)
        n143 = call "GL Set Operation Mode.vi"("position cts (abs/rel)"=w378, "Position Mode (Absolute)"=w371, "error in (no error)"=w381, "Start Now?"=TRUE, "Axis"=w375, "Galil.IGalil"=w376) -> ("error out"=w383:errorcluster)  [unwired: 3 in, 2 out]
      }
      event "W Position (mm)": Value Change {
        n144 = event-data() -> ("NewVal"=w398:dbl)  [unwired: 1 out]
        n145 = Multiply(x=w398, y=w397) -> (x*y=w393:dbl)
        n146 = Subtract(x=w393, y=0.0) -> ()  [unwired: 1 out]
        n147 = call "GL Set Operation Mode.vi"("position cts (abs/rel)"=w393, "Position Mode (Absolute)"=w391, "error in (no error)"=w389, "Start Now?"=TRUE, "Axis"=w394, "Galil.IGalil"=w392) -> ("error out"=w390:errorcluster)  [unwired: 3 in, 2 out]
      }
      event "Select V&A": Value Change {
        n148 = event-data() -> ()  [unwired: 2 out]
        n149 = call "GL_SetVandA.vi"("error in"=w399, "Motion Settings"=w402, "Refnum in"=w401) -> ("error out"=w404:errorcluster, "Motion Settings Out"=w400:T1)  [unwired: 6 in, 1 out]
        n150 = local write "Select V&A"(FALSE ("Select V&A")) -> ()
      }
      event Key Down {
        w412 = T11[] [enum."Up", enum."Down", enum."Left", enum."Right", enum."PageUp", enum."PageDown"] items=["ASCII", "Enter", "Return", "Shift", "Ctrl", "Alt", "Cmd", "Opt", "Caps", "NumLock", "Clear", "Break", "Up", "Down", "Left", "Right", "Insert", "Delete", "Home", "End", "PageUp", "PageDown", "Escape", "Help", "Pause", "ScrollLock", "F1", "F2", "F3", "F4", "F5", "F6", "F7", "F8", "F9", "F10", "F11", "F12", "F13", "F14", "F15", "F16", "F17", "F18", "F19", "F20", "F21", "F22", "F23", "F24", "Play", "VolumeUp", "VolumeDown", "Mute", "Two Byte Char"]
        n151 = event-data() -> ("VKey"=w414:T11, "Char"=w418:i16, "PlatMods"=w421:T12)  [unwired: 1 out]
        n152 = property on="Y Position (mm)" class="DigNum (strict)"() -> ("Key Focus"=w411:bool)  [unwired: 2 in, 2 out]
        n153 = property on="W Position (mm)" class="DigNum (strict)"() -> ("Key Focus"=w410:bool)  [unwired: 2 in, 2 out]
        n154 = property on="Z Position (mm)" class="DigNum (strict)"() -> ("Key Focus"=w409:bool)  [unwired: 2 in, 2 out]
        n155 = property on="X Position (mm)" class="DigNum (strict)"() -> ("Key Focus"=w408:bool)  [unwired: 2 in, 2 out]
        n156 = property on="Inc. Step\nSize (mm)" class="DigNum (strict)"() -> ("Key Focus"=w407:bool)  [unwired: 2 in, 2 out]
        n157 = Equal?(x=w418, y=i16[] [90, 122, 67, 99]) -> (x = y?=w416:bool[])
        n158 = Equal?(x=w414, y=w412) -> (x = y?=w419:bool[])
        n159 = Or Array Elements(Boolean array=w416) -> (logical OR=w415:bool)
        n160 = Or Array Elements(Boolean array=w419) -> (logical OR=w413:bool)
        n161 = Or(x=w415, y=w413) -> (x .or. y?=w406:bool)
        n162 = Compound Arithmetic op=OR(w411, w410, w409, w408, w407) -> (w405:bool)
        n163 = stacked-sequence {
          tunnel: "Axis Tune" -> [w425 _ _]
          tunnel: w422 -> [_ w437 _]
          tunnel: w421 -> [_ w436 _]
          tunnel: w414 -> [_ w435 _]
          tunnel: w418 -> [_ w434 _]
          tunnel: [_ w433 _] -> w420
          tunnel: w406 -> [w424 _ w441]
          tunnel: w405 -> [_ w432 _]
          frame #0 {
            n164 = case shown="True" w424 {
              tunnel: w425 -> [_ w427]
              frame False {
              }
              frame True {
                n165 = case shown="\"Axis 2\"" w427 {
                  tunnel: [w428 w429 w430 w431] -> w426
                  frame "Axis 1", Default {
                    n166 = property on="X Position (mm)" class="DigNum (strict)"() -> ("Value"=w428:dbl)  [unwired: 2 in, 2 out]
                  }
                  frame "Axis 2" {
                    n167 = property on="Y Position (mm)" class="DigNum (strict)"() -> ("Value"=w429:dbl)  [unwired: 2 in, 2 out]
                  }
                  frame "Axis 3" {
                    n168 = property on="Z Position (mm)" class="DigNum (strict)"() -> ("Value"=w430:dbl)  [unwired: 2 in, 2 out]
                  }
                  frame "Axis 4" {
                    n169 = property on="W Position (mm)" class="DigNum (strict)"() -> ("Value"=w431:dbl)  [unwired: 2 in, 2 out]
                  }
                }
                n170 = property on="Position (mm) (Abs)" class="DigNum (strict)"("Value"=w426) -> ()  [unwired: 2 in, 2 out]
              }
            }
          }
          frame #1 {
            n171 = control-ref of="Axis Tune"() -> (w439:refnum<vi>)
            n172 = control-ref of="Position (mm) (Abs)"() -> (w440:refnum<vi>)
            n173 = call "KeyboardNudge.vi"("Axis Tune Refnum"=w439, "Char"=w434, "Position (mm) Refnum"=w440, "Ignore Key Down"=w432, "VKey"=w435, "PlatMods"=w436, "Inc. Step Size (mm)"="Inc. Step\nSize (mm)", "Motion Settings"=w437) -> ("Quit"=w433:bool)  [unwired: 10 in, 1 out]
          }
          frame #2 {
            n174 = case shown="True" w441 {
              frame False {
              }
              frame True {
                n175 = property on="Axis Tune" class="RadioBtnsControl (strict)"() -> ("Value"=w442:enum32{"Axis 1", "Axis 2", "Axis 3", "Axis 4"})  [unwired: 2 in, 2 out]
                n176 = case shown="\"Axis 1\", Default" w442 {
                  tunnel: "Position (mm) (Abs)" -> [w444 w445 w446 w447]
                  frame "Axis 1", Default {
                    n177 = property on="X Position (mm)" class="DigNum (strict)"("Val(Sgnl)"=w444) -> ()  [unwired: 2 in, 2 out]
                  }
                  frame "Axis 2" {
                    n178 = property on="Y Position (mm)" class="DigNum (strict)"("Val(Sgnl)"=w445) -> ()  [unwired: 2 in, 2 out]
                  }
                  frame "Axis 3" {
                    n179 = property on="Z Position (mm)" class="DigNum (strict)"("Val(Sgnl)"=w446) -> ()  [unwired: 2 in, 2 out]
                  }
                  frame "Axis 4" {
                    n180 = property on="W Position (mm)" class="DigNum (strict)"("Val(Sgnl)"=w447) -> ()  [unwired: 2 in, 2 out]
                  }
                }
              }
            }
          }
        }
      }
      event "Cent X": Value Change {
        n181 = event-data() -> ("CtlRef"=w456:refnum<vi>)  [unwired: 1 out]
        n182 = Unbundle By Name(w450) -> ("Motion Profile"=w449:string)
        n183 = Two Button Dialog(message=w453) -> (T button?=w452:bool)  [unwired: 2 in]
        n184 = case shown="True" w452 {
          tunnel: w451 -> [_ w462]
          tunnel: w456 -> [_ w461]
          tunnel: w455 -> [_ w460]
          tunnel: w454 -> [_ w459]
          tunnel: w449 -> [_ w458]
          tunnel: w448 -> [_ w457]
          frame False {
          }
          frame True {
            n185 = case shown="\"False\", Default" w458 {
              tunnel: w462 -> [w468 w477]
              tunnel: w461 -> [w475 _]
              tunnel: w460 -> [w474 w479]
              tunnel: w459 -> [w471 _]
              tunnel: w457 -> [w464 w478]
              frame "False", Default {
                w466 = TRUE
                n186 = Not(x=w466) -> (.not. x?=w469:bool)
                n187 = property on="Property Node" class="Bool"(reference=w475, error in=w474, "Blinking"=w466) -> (reference out=w472:refnum<vi>, error out=w463:errorcluster)
                n188 = property class="Bool (strict)"(reference=w471, "Value"=w469) -> (reference out=w470:refnum<vi>)  [unwired: 1 in, 1 out]
                n189 = call "GL Center.vi"("error in"=w463, "Axis"=w468, "Galil.IGalil"=w464) -> ("error out"=w465:errorcluster)  [unwired: 4 in, 2 out]
                n190 = property on="Property Node" class="Bool"(reference=w472, error in=w465, "Blinking"=FALSE) -> (error out=w467:errorcluster)  [unwired: 1 out]
                n191 = property class="Bool (strict)"(reference=w470, error in=w467, "Value"=w466) -> ()  [unwired: 2 out]
              }
              frame "XY_Stage" {
                n192 = call "GL_HomeSWLims.vi"("SoftwareLims?"=TRUE, "error in"=w479, "Axis IN"=w477, "Galil.IGalil"=w478) -> ()  [unwired: 5 in, 3 out]
              }
            }
          }
        }
      }
      event "Cent Y": Value Change {
        n193 = event-data() -> ("CtlRef"=w488:refnum<vi>)  [unwired: 1 out]
        n194 = Two Button Dialog(message=w485) -> (T button?=w484:bool)  [unwired: 2 in]
        n195 = Unbundle By Name(w483) -> ("Motion Profile"=w482:string)
        n196 = case shown="True" w484 {
          tunnel: w489 -> [_ w493]
          tunnel: w488 -> [_ w496]
          tunnel: TRUE -> [_ w495]
          tunnel: w486 -> [_ w494]
          tunnel: w482 -> [_ w492]
          tunnel: w481 -> [_ w491]
          tunnel: w480 -> [_ w490]
          frame False {
          }
          frame True {
            n197 = case shown="\"XY_Stage\"" w492 {
              tunnel: w496 -> [_ w511]
              tunnel: w495 -> [_ w501]
              tunnel: w494 -> [_ w509]
              tunnel: w493 -> [w499 w504]
              tunnel: w491 -> [w500 w505]
              tunnel: w490 -> [w497 _]
              frame "XY_Stage" {
                n198 = call "GL_HomeSWLims.vi"("SoftwareLims?"=TRUE, "error in"=w497, "Axis IN"=w499, "Galil.IGalil"=w500) -> ()  [unwired: 5 in, 3 out]
              }
              frame "True", Default {
                n199 = Not(x=w501) -> (.not. x?=w510:bool)
                n200 = property on="Property Node" class="Bool"(reference=w511, "Blinking"=w501) -> (reference out=w507:refnum<vi>, error out=w506:errorcluster)  [unwired: 1 in]
                n201 = property class="Bool (strict)"(reference=w509, "Value"=w510) -> (reference out=w508:refnum<vi>)  [unwired: 1 in, 1 out]
                n202 = call "GL Center.vi"("error in"=w506, "Axis"=w504, "Galil.IGalil"=w505) -> ("error out"=w503:errorcluster)  [unwired: 4 in, 2 out]
                n203 = property on="Property Node" class="Bool"(reference=w507, error in=w503, "Blinking"=FALSE) -> (error out=w502:errorcluster)  [unwired: 1 out]
                n204 = property class="Bool (strict)"(reference=w508, error in=w502, "Value"=w501) -> ()  [unwired: 2 out]
              }
            }
          }
        }
      }
      event "Cent Z": Value Change {
        n205 = event-data() -> ("CtlRef"=w518:refnum<vi>)  [unwired: 1 out]
        n206 = Two Button Dialog(message=w515) -> (T button?=w516:bool)  [unwired: 2 in]
        n207 = case shown="False" w516 {
          tunnel: w519 -> [_ w522]
          tunnel: w518 -> [_ w530]
          tunnel: w517 -> [_ w529]
          tunnel: w514 -> [_ w521]
          tunnel: w513 -> [_ _]
          frame False {
          }
          frame True {
            w524 = TRUE
            n208 = property on="Property Node" class="Bool"(reference=w530, "Blinking"=w524) -> (reference out=w531:refnum<vi>, error out=w525:errorcluster)  [unwired: 1 in]
            n209 = Not(x=w524) -> (.not. x?=w527:bool)
            n210 = property class="Bool (strict)"(reference=w529, "Value"=w527) -> (reference out=w528:refnum<vi>)  [unwired: 1 in, 1 out]
            n211 = call "GL Center.vi"("Simple"=TRUE, "error in"=w525, "Axis"=w522, "Galil.IGalil"=w521) -> ("error out"=w526:errorcluster)  [unwired: 3 in, 2 out]
            n212 = property on="Property Node" class="Bool"(reference=w531, error in=w526, "Blinking"=FALSE) -> (error out=w523:errorcluster)  [unwired: 1 out]
            n213 = property class="Bool (strict)"(reference=w528, error in=w523, "Value"=w524) -> ()  [unwired: 2 out]
          }
        }
      }
      event "Cent W": Value Change {
        w536 = TRUE
        # "Center the motion stage"
        n214 = event-data() -> ("CtlRef"=w544:refnum<vi>)  [unwired: 1 out]
        n215 = Not(x=w536) -> (.not. x?=w542:bool)
        n216 = property on="Property Node" class="Bool"(reference=w544, error in=w538, "Blinking"=w536) -> (reference out=w545:refnum<vi>, error out=w535:errorcluster)
        n217 = property class="Bool (strict)"(reference=w543, "Value"=w542) -> (reference out=w541:refnum<vi>)  [unwired: 1 in, 1 out]
        n218 = call "GL Center.vi"("error in"=w535, "Axis"=w539, "Galil.IGalil"=w540) -> ("error out"=w537:errorcluster)  [unwired: 4 in, 2 out]
        n219 = property on="Property Node" class="Bool"(reference=w545, error in=w537, "Blinking"=FALSE) -> (error out=w534:errorcluster)  [unwired: 1 out]
        n220 = property class="Bool (strict)"(reference=w541, error in=w534, "Value"=w536) -> ()  [unwired: 2 out]
      }
      event "Cent All": Value Change {
        n221 = event-data() -> ("CtlRef"=w553:refnum<vi>)  [unwired: 1 out]
        n222 = Unbundle By Name(w551) -> ("Motion Profile"=w550:string)
        n223 = case shown="\"True\", Default" w550 {
          tunnel: w553 -> [_ w564]
          tunnel: w552 -> [_ w563]
          tunnel: w551 -> [_ _]
          tunnel: w549 -> [_ w556]
          tunnel: w548 -> [_ w555]
          tunnel: w547 -> [_ w554]
          frame "XY_Stage" {
          }
          frame "True", Default {
            w557 = TRUE
            # "Center the motion stage"
            n224 = property on="Property Node" class="Bool"(reference=w564, error in=w554, "Blinking"=w557) -> (reference out=w565:refnum<vi>, error out=w559:errorcluster)
            n225 = Not(x=w557) -> (.not. x?=w562:bool)
            n226 = for {
              N: w555 -> [_]
              tunnel: w556 -> [w568]
              shift-right: [w569] -> w558
              shift-left: w559 -> [w570]
              i -> [w567]
              n227 = call "GL Center.vi"("error in"=w570, "Axis"=w567, "Galil.IGalil"=w568) -> ("error out"=w569:errorcluster)  [unwired: 4 in, 2 out]
            }
            n228 = property class="Bool (strict)"(reference=w563, "Value"=w562) -> (reference out=w561:refnum<vi>)  [unwired: 1 in, 1 out]
            n229 = property on="Property Node" class="Bool"(reference=w565, error in=w558, "Blinking"=FALSE) -> (error out=w560:errorcluster)  [unwired: 1 out]
            n230 = property class="Bool (strict)"(reference=w561, error in=w560, "Value"=w557) -> ()  [unwired: 2 out]
          }
        }
      }
      event "Ratio Num", "Ratio Denom", "Master Axis", "Slave Axis": Value Change {
        (unwired) TRUE ("Gearing (Absolute)")
        # "Set up master slave motion."
        n231 = event-data() -> ()  [unwired: 2 out]
        n232 = Divide(x="Ratio Num", y="Ratio Denom") -> (x/y=w574:dbl)
        n233 = expression code="atan(x)*360/2/3.14159"(w574) -> (→"Angle":dbl)
      }
      event "Enable Gearing": Value Change {
        # "Slave axis 2 to motion."
        n234 = event-data() -> ()  [unwired: 2 out]
      }
      event "Def Abs": Value Change {
        # "Display controls for updating global locations"
        n235 = event-data() -> ("NewVal"=w577:bool)  [unwired: 3 out]
        n236 = case shown="False" w577 {
          tunnel: [T7."Disabled and Grayed Out" ("Disabled") T7."Enabled" ("Disabled")] -> w578
          frame False {
          }
          frame True {
          }
        }
        n237 = property on="Abs X Pos (mm)" class="DigNum (strict)"("DisabledEnum"=w578) -> ()  [unwired: 2 in, 2 out]
        n238 = property on="Abs Y Pos (mm)" class="DigNum (strict)"("DisabledEnum"=w578) -> ()  [unwired: 2 in, 2 out]
        n239 = property on="Abs Z Pos (mm)" class="DigNum (strict)"("DisabledEnum"=w578) -> ()  [unwired: 2 in, 2 out]
        n240 = property on="Abs W Pos (mm)" class="DigNum (strict)"("DisabledEnum"=w578) -> ()  [unwired: 2 in, 2 out]
      }
      event "Abs X Pos (mm)": Value Change {
        # "Update global value and hide indicator.\nNew value will be reflected in position feedback."
        n241 = event-data() -> ()  [unwired: 2 out]
        n242 = Multiply(x=w590, y="Abs X Pos (mm)") -> (x*y=w583:dbl)
        n243 = call "GL Command Set.vi"("Command"=Command_Menu."Define Pos", "error in (no error)"=w585, "Value"=w583, "Axis"=w584, "Galil.IGalil"=w582) -> ("error out"=w586:errorcluster)  [unwired: 2 in, 4 out]
      }
      event "Abs Y Pos (mm)": Value Change {
        # "Update global value and hide indicator.\nNew value will be reflected in position feedback."
        n244 = event-data() -> ()  [unwired: 2 out]
        n245 = Multiply(x=w598, y="Abs Y Pos (mm)") -> (x*y=w594:dbl)
        n246 = call "GL Command Set.vi"("Command"=Command_Menu."Define Pos", "error in (no error)"=w591, "Value"=w594, "Axis"=w593) -> ("error out"=w592:errorcluster)  [unwired: 3 in, 4 out]
      }
      event "Abs Z Pos (mm)": Value Change {
        # "Update global value and hide indicator.\nNew value will be reflected in position feedback."
        n247 = event-data() -> ()  [unwired: 2 out]
        n248 = Multiply(x=w609, y="Abs Z Pos (mm)") -> (x*y=w608:dbl)
        n249 = Multiply(x=w608, y=w607) -> (x*y=w602:dbl)
        n250 = call "GL Command Set.vi"("Command"=Command_Menu."Define Pos", "error in (no error)"=w599, "Value"=w602, "Axis"=w603, "Galil.IGalil"=w601) -> ("error out"=w600:errorcluster)  [unwired: 2 in, 4 out]
      }
      event "Abs W Pos (mm)": Value Change {
        # "Update global value and hide indicator.\nNew value will be reflected in position feedback."
        n251 = event-data() -> ()  [unwired: 2 out]
        n252 = Multiply(x=w618, y="Abs W Pos (mm)") -> (x*y=w612:dbl)
        n253 = call "GL Command Set.vi"("Command"=Command_Menu."Define Pos", "error in (no error)"=w613, "Value"=w612, "Axis"=w610, "Galil.IGalil"=w611) -> ("error out"=w614:errorcluster)  [unwired: 2 in, 4 out]
      }
    }
    n254 = Unbundle By Name(w82) -> ("status"=w73:bool)
    n255 = Compound Arithmetic op=OR(w73, "stop", w71) -> (w86:bool)
  }
  "error out" <- w14
  n256 = call "FindLocation.vi"("Motion Settings"=w10) -> ("Motion Settings Out"=w3:T1, "error out"=w6:errorcluster)  [unwired: 2 in, 2 out]
  "Motion Settings Out" <- w3
  n257 = Unbundle By Name(w3) -> ("GL Ref Out"=w2:refnum<k7>)
  n258 = call "GL Command Set.vi"("Command"=Command_Menu."Motor Off", "error in (no error)"=w6, "Axis"=w1, "Galil.IGalil"=w2) -> ()  [unwired: 3 in, 5 out]
